vi "START SEARCH DATABASE.vi"(11 "REFERENCES":T1) -> ()   [LabVIEW 2019]
uses:
  Controls/References Cluster.ctl
  Controls/Custom Calendar/Custom Calendar.xctl
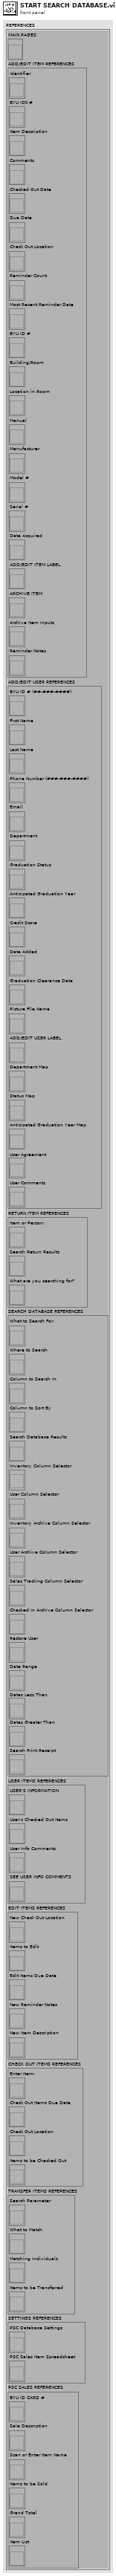
[diagram p1: front panel]
types:
  T1 = typedef "References Cluster.ctl" = cluster{"MAIN PAGES":refnum<vi>, "ADD/EDIT ITEM REFERENCES":cluster{"Identifier":refnum<vi>, "BYU ICN #":refnum<vi>, "Item Description":refnum<vi>, "Comments":refnum<vi>, "Checked Out Date":refnum<vi>, "Due Date":refnum<vi>, "Check Out Location":refnum<vi>, "Reminder Count":refnum<vi>, "Most Recent Reminder Date":refnum<vi>, "BYU ID #":refnum<vi>, "Building/Room":refnum<vi>, "Location in Room":refnum<vi>, "Manual":refnum<vi>, "Manufacturer":refnum<vi>, "Model #":refnum<vi>, "Serial #":refnum<vi>, "Date Acquired":refnum<vi>, "ADD/EDIT ITEM LABEL":refnum<vi>, "ARCHIVE ITEM":refnum<vi>, "Archive Item Inputs":refnum<vi>, "Reminder Notes":refnum<vi>}, "ADD/EDIT USER REFERENCES":cluster{"BYU ID # (##-###-####)":refnum<vi>, "First Name":refnum<vi>, "Last Name":refnum<vi>, "Phone Number (###-###-####)":refnum<vi>, "Email":refnum<vi>, "Department":refnum<vi>, "Graduation Status":refnum<vi>, "Anticipated Graduation Year":refnum<vi>, "Credit Score":refnum<vi>, "Date Added":refnum<vi>, "Graduation Clearance Date":refnum<vi>, "Picture File Name":refnum<vi>, "ADD/EDIT USER LABEL":refnum<vi>, "Department Map":refnum<vi>, "Status Map":refnum<vi>, "Anticipated Graduation Year Map":refnum<vi>, "User Agreement":refnum<vi>, "User Comments":refnum<vi>}, "RETURN ITEM REFERENCES":cluster{"Item or Person:":refnum<vi>, "Search Return Results":refnum<vi>, "What are you searching for?":refnum<vi>}, "SEARCH DATABASE REFERENCES":cluster{"What to Search For:":refnum<vi>, "Where to Search":refnum<vi>, "Column to Search In":refnum<vi>, "Column to Sort By":refnum<vi>, "Search Database Results":refnum<vi>, "Inventory Column Selector":refnum<vi>, "User Column Selector":refnum<vi>, "Inventory Archive Column Selector":refnum<vi>, "User Archive Column Selector":refnum<vi>, "Sales Tracking Column Selector":refnum<vi>, "Checked In Archive Column Selector":refnum<vi>, "Restore User":refnum<vi>, "Date Range":refnum<vi>, "Dates Less Than":refnum<vi>, "Dates Greater Than":refnum<vi>, "Search Print Receipt":refnum<vi>}, "USER ITEMS REFERENCES":cluster{"USER'S INFORMATION":refnum<vi>, "User's Checked Out Items":refnum<vi>, "User Info Comments":refnum<vi>, "SEE USER INFO COMMENTS":refnum<vi>}, "EDIT ITEMS REFERENCES":cluster{"New Check Out Location":refnum<vi>, "Items to Edit":refnum<vi>, "Edit Items Due Date":refnum<vi>, "New Reminder Notes":refnum<vi>, "New Item Description":refnum<vi>}, "CHECK OUT ITEMS REFERENCES":cluster{"Enter Item:":refnum<vi>, "Check Out Items Due Date":refnum<vi>, "Check Out Location":refnum<vi>, "Items to be Checked Out":refnum<vi>}, "TRANSFER ITEMS REFERENCES":cluster{"Search Parameter":refnum<vi>, "What to Match":refnum<vi>, "Matching Individuals":refnum<vi>, "Items to be Transferred":refnum<vi>}, "SETTINGS REFERENCES":cluster{"PSC Database Settings":refnum<vi>, "PSC Sales Item Spreadsheet":refnum<vi>}, "PSC SALES REFERENCES":cluster{"BYU ID CARD #":refnum<vi>, "Sale Description":refnum<vi>, "Scan or Enter Item Name":refnum<vi>, "Items to be Sold":refnum<vi>, "Grand Total":refnum<vi>, "Item List":refnum<vi>}}
  T2 = cluster{"What to Search For:":refnum<vi>, "Where to Search":refnum<vi>, "Column to Search In":refnum<vi>, "Column to Sort By":refnum<vi>, "Search Database Results":refnum<vi>, "Inventory Column Selector":refnum<vi>, "User Column Selector":refnum<vi>, "Inventory Archive Column Selector":refnum<vi>, "User Archive Column Selector":refnum<vi>, "Sales Tracking Column Selector":refnum<vi>, "Checked In Archive Column Selector":refnum<vi>, "Restore User":refnum<vi>, "Date Range":refnum<vi>, "Dates Less Than":refnum<vi>, "Dates Greater Than":refnum<vi>, "Search Print Receipt":refnum<vi>}
  T3 = enum32{"IDLE", "ADD/EDIT USER", "ADD/EDIT ITEM", "RETURN ITEMS", "SEARCH DATABASE", "USER ITEMS", "CHECK OUT ITEMS", "EDIT ITEMS", "TRANSFER ITEMS", "PSC SALES", "ATRIUM", "INVENTORY TRACKING", "SETTINGS"}
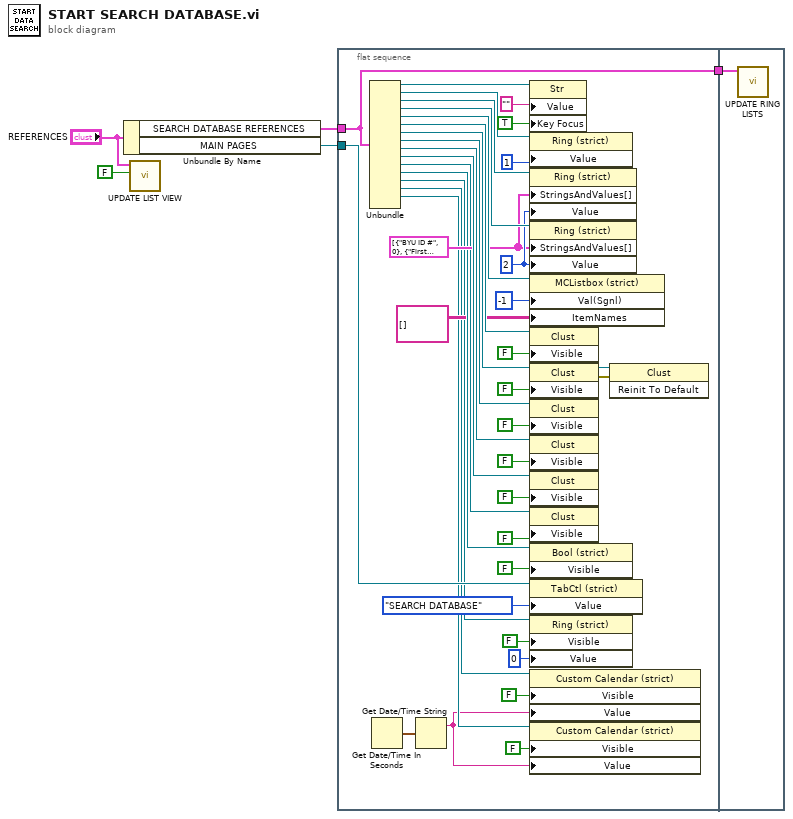
[diagram p0: block diagram]
diagram:
  n1 = Unbundle By Name("REFERENCES") -> ("SEARCH DATABASE REFERENCES"=w4:T2, "MAIN PAGES"=w1:refnum<vi>)
  n2 = call "UPDATE LIST VIEW.vi"("COLUMNS TO VIEW"=FALSE, "REFERENCES"="REFERENCES") -> ()  [unwired: 10 in]
  n3 = flat-sequence {
    tunnel: w4 -> [w26]
    tunnel: [w26] -> w5
    tunnel: w1 -> [w24]
    tunnel: w5 -> [w46]
    frame #0 {
      w25 = cluster{"String":string, "Value":u16}[] [{"String"="BYU ID #", "Value"=0}, {"String"="First Name", "Value"=1}, {"String"="Last Name", "Value"=2}, {"String"="Phone Number", "Value"=3}, {"String"="Email", "Value"=4}, {"String"="Department", "Value"=5}, {"String"="Graduation Status", "Value"=6}, {"String"="Anticipated Graduation Year", "Value"=7}, {"String"="Credit Score", "Value"=8}, {"String"="Date Added", "Value"=9}, {"String"="Graduation Clearance Date", "Value"=10}, {"String"="Profile Picture Path", "Value"=11}] ("Strings And Values []")
      w28 = u16 2 ("Value")
      n4 = Unbundle(w26) -> ("What to Search For:"=w45:refnum<vi>, "Where to Search"=w44:refnum<vi>, "Column to Search In"=w43:refnum<vi>, "Column to Sort By"=w42:refnum<vi>, "Search Database Results"=w41:refnum<vi>, "Inventory Column Selector"=w34:refnum<vi>, "User Column Selector"=w40:refnum<vi>, "Inventory Archive Column Selector"=w39:refnum<vi>, "User Archive Column Selector"=w38:refnum<vi>, "Sales Tracking Column Selector"=w37:refnum<vi>, "Checked In Archive Column Selector"=w21:refnum<vi>, "Restore User"=w19:refnum<vi>, "Date Range"=w14:refnum<vi>, "Dates Less Than"=w13:refnum<vi>, "Dates Greater Than"=w12:refnum<vi>)  [unwired: 1 out]
      n5 = Get Date/Time In Seconds() -> (seconds since 1Jan1904=w7:timestamp)
      n6 = Get Date/Time String(seconds (now)=w7) -> (date string=w6:string)  [unwired: 2 in, 1 out]
      n7 = property class="Str"(reference=w45, "Value"="", "Key Focus"=TRUE) -> ()  [unwired: 1 in, 2 out]
      n8 = property class="Ring (strict)"(reference=w44, "Value"=u16 1) -> ()  [unwired: 1 in, 2 out]
      n9 = property class="Ring (strict)"(reference=w43, "StringsAndValues[]"=w25, "Value"=w28) -> ()  [unwired: 1 in, 2 out]
      n10 = property class="Ring (strict)"(reference=w42, "StringsAndValues[]"=w25, "Value"=w28) -> ()  [unwired: 1 in, 2 out]
      n11 = property class="MCListbox (strict)"(reference=w41, "Val(Sgnl)"=-1 ("Value"), "ItemNames"=string[][] [] ("Item Names")) -> ()  [unwired: 1 in, 2 out]
      n12 = property class="Clust"(reference=w34, "Visible"=FALSE) -> ()  [unwired: 1 in, 2 out]
      n13 = property class="Clust"(reference=w40, "Visible"=FALSE) -> (reference out=w16:refnum<vi>, error out=w15:errorcluster)  [unwired: 1 in]
      n14 = property class="Clust"(reference=w39, "Visible"=FALSE) -> ()  [unwired: 1 in, 2 out]
      n15 = property class="Clust"(reference=w38, "Visible"=FALSE) -> ()  [unwired: 1 in, 2 out]
      n16 = property class="Clust"(reference=w37, "Visible"=FALSE) -> ()  [unwired: 1 in, 2 out]
      n17 = property class="Clust"(reference=w21, "Visible"=FALSE) -> ()  [unwired: 1 in, 2 out]
      n18 = property class="Bool (strict)"(reference=w19, "Visible"=FALSE) -> ()  [unwired: 1 in, 2 out]
      n19 = property class="TabCtl (strict)"(reference=w24, "Value"=T3."SEARCH DATABASE") -> ()  [unwired: 1 in, 2 out]
      n20 = property class="Ring (strict)"(reference=w14, "Visible"=FALSE, "Value"=u16 0) -> ()  [unwired: 1 in, 2 out]
      n21 = property class="Custom Calendar (strict)"(reference=w13, "Visible"=FALSE, "Value"=w6) -> ()  [unwired: 1 in, 2 out]
      n22 = property class="Custom Calendar (strict)"(reference=w12, "Visible"=FALSE, "Value"=w6) -> ()  [unwired: 1 in, 2 out]
      n23 = invoke class="Clust" method="Reinit To Default"(reference=w16, error in=w15) -> ()  [unwired: 1 in, 3 out]
    }
    frame #1 {
      n24 = call "UPDATE RING LISTS.vi"("SEARCH DATABASE REFERENCES"=w46) -> ()  [unwired: 11 in]
    }
  }
